vi "PCO_FW_Vers.vi"() -> (0 "PCO_FW_Vers":T2, 1 "PCO_FW_Vers_Raw":T1, 2 "Length":u16, 3 "Raw_Length":u16)   [LabVIEW 2020, in "SDK.lvlib" / "Structures.lvlib"]
doc: "Use this template to build a VI to use as a subVI."
uses:
  Structures.lvlib
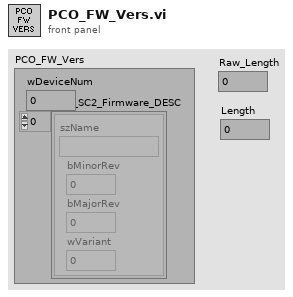
[diagram p1: front panel]
types:
  T1 = cluster{"wDeviceNum":u16, "PCO_SC2_Firmware_DESC":cluster{"PCO_SC2_FW_Desc_Raw":cluster{"szName":cluster{u8, u8, u8, u8, u8, u8, u8, u8, u8, u8, u8, u8, u8, u8, u8, u8}, "bMinorRev":u8, "bMajorRev":u8, "wVariant":u16, "zzwDummy":cluster{u16, u16, u16, u16, u16, u16, u16, u16, u16, u16, u16, u16, u16, u16, u16, u16, u16, u16, u16, u16, u16, u16}}, "PCO_SC2_FW_Desc_Raw":cluster{"szName":cluster{u8, u8, u8, u8, u8, u8, u8, u8, u8, u8, u8, u8, u8, u8, u8, u8}, "bMinorRev":u8, "bMajorRev":u8, "wVariant":u16, "zzwDummy":cluster{u16, u16, u16, u16, u16, u16, u16, u16, u16, u16, u16, u16, u16, u16, u16, u16, u16, u16, u16, u16, u16, u16}}, "PCO_SC2_FW_Desc_Raw":cluster{"szName":cluster{u8, u8, u8, u8, u8, u8, u8, u8, u8, u8, u8, u8, u8, u8, u8, u8}, "bMinorRev":u8, "bMajorRev":u8, "wVariant":u16, "zzwDummy":cluster{u16, u16, u16, u16, u16, u16, u16, u16, u16, u16, u16, u16, u16, u16, u16, u16, u16, u16, u16, u16, u16, u16}}, "PCO_SC2_FW_Desc_Raw":cluster{"szName":cluster{u8, u8, u8, u8, u8, u8, u8, u8, u8, u8, u8, u8, u8, u8, u8, u8}, "bMinorRev":u8, "bMajorRev":u8, "wVariant":u16, "zzwDummy":cluster{u16, u16, u16, u16, u16, u16, u16, u16, u16, u16, u16, u16, u16, u16, u16, u16, u16, u16, u16, u16, u16, u16}}, "PCO_SC2_FW_Desc_Raw":cluster{"szName":cluster{u8, u8, u8, u8, u8, u8, u8, u8, u8, u8, u8, u8, u8, u8, u8, u8}, "bMinorRev":u8, "bMajorRev":u8, "wVariant":u16, "zzwDummy":cluster{u16, u16, u16, u16, u16, u16, u16, u16, u16, u16, u16, u16, u16, u16, u16, u16, u16, u16, u16, u16, u16, u16}}, "PCO_SC2_FW_Desc_Raw":cluster{"szName":cluster{u8, u8, u8, u8, u8, u8, u8, u8, u8, u8, u8, u8, u8, u8, u8, u8}, "bMinorRev":u8, "bMajorRev":u8, "wVariant":u16, "zzwDummy":cluster{u16, u16, u16, u16, u16, u16, u16, u16, u16, u16, u16, u16, u16, u16, u16, u16, u16, u16, u16, u16, u16, u16}}, "PCO_SC2_FW_Desc_Raw":cluster{"szName":cluster{u8, u8, u8, u8, u8, u8, u8, u8, u8, u8, u8, u8, u8, u8, u8, u8}, "bMinorRev":u8, "bMajorRev":u8, "wVariant":u16, "zzwDummy":cluster{u16, u16, u16, u16, u16, u16, u16, u16, u16, u16, u16, u16, u16, u16, u16, u16, u16, u16, u16, u16, u16, u16}}, "PCO_SC2_FW_Desc_Raw":cluster{"szName":cluster{u8, u8, u8, u8, u8, u8, u8, u8, u8, u8, u8, u8, u8, u8, u8, u8}, "bMinorRev":u8, "bMajorRev":u8, "wVariant":u16, "zzwDummy":cluster{u16, u16, u16, u16, u16, u16, u16, u16, u16, u16, u16, u16, u16, u16, u16, u16, u16, u16, u16, u16, u16, u16}}, "PCO_SC2_FW_Desc_Raw":cluster{"szName":cluster{u8, u8, u8, u8, u8, u8, u8, u8, u8, u8, u8, u8, u8, u8, u8, u8}, "bMinorRev":u8, "bMajorRev":u8, "wVariant":u16, "zzwDummy":cluster{u16, u16, u16, u16, u16, u16, u16, u16, u16, u16, u16, u16, u16, u16, u16, u16, u16, u16, u16, u16, u16, u16}}, "PCO_SC2_FW_Desc_Raw":cluster{"szName":cluster{u8, u8, u8, u8, u8, u8, u8, u8, u8, u8, u8, u8, u8, u8, u8, u8}, "bMinorRev":u8, "bMajorRev":u8, "wVariant":u16, "zzwDummy":cluster{u16, u16, u16, u16, u16, u16, u16, u16, u16, u16, u16, u16, u16, u16, u16, u16, u16, u16, u16, u16, u16, u16}}}}
  T2 = cluster{"wDeviceNum":u16, "PCO_SC2_Firmware_DESC":cluster{"szName":string, "bMinorRev":u8, "bMajorRev":u8, "wVariant":u16}[]}
  T3 = cluster{"szName":string, "bMinorRev":u8, "bMajorRev":u8, "wVariant":u16}
  T4 = cluster{"szName":cluster{u8, u8, u8, u8, u8, u8, u8, u8, u8, u8, u8, u8, u8, u8, u8, u8}, "bMinorRev":u8, "bMajorRev":u8, "wVariant":u16, "zzwDummy":cluster{u16, u16, u16, u16, u16, u16, u16, u16, u16, u16, u16, u16, u16, u16, u16, u16, u16, u16, u16, u16, u16, u16}}
  T5 = cluster{"PCO_SC2_FW_Desc_Raw":cluster{"szName":cluster{u8, u8, u8, u8, u8, u8, u8, u8, u8, u8, u8, u8, u8, u8, u8, u8}, "bMinorRev":u8, "bMajorRev":u8, "wVariant":u16, "zzwDummy":cluster{u16, u16, u16, u16, u16, u16, u16, u16, u16, u16, u16, u16, u16, u16, u16, u16, u16, u16, u16, u16, u16, u16}}, "PCO_SC2_FW_Desc_Raw":cluster{"szName":cluster{u8, u8, u8, u8, u8, u8, u8, u8, u8, u8, u8, u8, u8, u8, u8, u8}, "bMinorRev":u8, "bMajorRev":u8, "wVariant":u16, "zzwDummy":cluster{u16, u16, u16, u16, u16, u16, u16, u16, u16, u16, u16, u16, u16, u16, u16, u16, u16, u16, u16, u16, u16, u16}}, "PCO_SC2_FW_Desc_Raw":cluster{"szName":cluster{u8, u8, u8, u8, u8, u8, u8, u8, u8, u8, u8, u8, u8, u8, u8, u8}, "bMinorRev":u8, "bMajorRev":u8, "wVariant":u16, "zzwDummy":cluster{u16, u16, u16, u16, u16, u16, u16, u16, u16, u16, u16, u16, u16, u16, u16, u16, u16, u16, u16, u16, u16, u16}}, "PCO_SC2_FW_Desc_Raw":cluster{"szName":cluster{u8, u8, u8, u8, u8, u8, u8, u8, u8, u8, u8, u8, u8, u8, u8, u8}, "bMinorRev":u8, "bMajorRev":u8, "wVariant":u16, "zzwDummy":cluster{u16, u16, u16, u16, u16, u16, u16, u16, u16, u16, u16, u16, u16, u16, u16, u16, u16, u16, u16, u16, u16, u16}}, "PCO_SC2_FW_Desc_Raw":cluster{"szName":cluster{u8, u8, u8, u8, u8, u8, u8, u8, u8, u8, u8, u8, u8, u8, u8, u8}, "bMinorRev":u8, "bMajorRev":u8, "wVariant":u16, "zzwDummy":cluster{u16, u16, u16, u16, u16, u16, u16, u16, u16, u16, u16, u16, u16, u16, u16, u16, u16, u16, u16, u16, u16, u16}}, "PCO_SC2_FW_Desc_Raw":cluster{"szName":cluster{u8, u8, u8, u8, u8, u8, u8, u8, u8, u8, u8, u8, u8, u8, u8, u8}, "bMinorRev":u8, "bMajorRev":u8, "wVariant":u16, "zzwDummy":cluster{u16, u16, u16, u16, u16, u16, u16, u16, u16, u16, u16, u16, u16, u16, u16, u16, u16, u16, u16, u16, u16, u16}}, "PCO_SC2_FW_Desc_Raw":cluster{"szName":cluster{u8, u8, u8, u8, u8, u8, u8, u8, u8, u8, u8, u8, u8, u8, u8, u8}, "bMinorRev":u8, "bMajorRev":u8, "wVariant":u16, "zzwDummy":cluster{u16, u16, u16, u16, u16, u16, u16, u16, u16, u16, u16, u16, u16, u16, u16, u16, u16, u16, u16, u16, u16, u16}}, "PCO_SC2_FW_Desc_Raw":cluster{"szName":cluster{u8, u8, u8, u8, u8, u8, u8, u8, u8, u8, u8, u8, u8, u8, u8, u8}, "bMinorRev":u8, "bMajorRev":u8, "wVariant":u16, "zzwDummy":cluster{u16, u16, u16, u16, u16, u16, u16, u16, u16, u16, u16, u16, u16, u16, u16, u16, u16, u16, u16, u16, u16, u16}}, "PCO_SC2_FW_Desc_Raw":cluster{"szName":cluster{u8, u8, u8, u8, u8, u8, u8, u8, u8, u8, u8, u8, u8, u8, u8, u8}, "bMinorRev":u8, "bMajorRev":u8, "wVariant":u16, "zzwDummy":cluster{u16, u16, u16, u16, u16, u16, u16, u16, u16, u16, u16, u16, u16, u16, u16, u16, u16, u16, u16, u16, u16, u16}}, "PCO_SC2_FW_Desc_Raw":cluster{"szName":cluster{u8, u8, u8, u8, u8, u8, u8, u8, u8, u8, u8, u8, u8, u8, u8, u8}, "bMinorRev":u8, "bMajorRev":u8, "wVariant":u16, "zzwDummy":cluster{u16, u16, u16, u16, u16, u16, u16, u16, u16, u16, u16, u16, u16, u16, u16, u16, u16, u16, u16, u16, u16, u16}}}
  T6 = cluster{"szName":string, "bMinorRev":u8, "bMajorRev":u8, "wVariant":u16}[]
  T7 = cluster{"wDeviceNum":u16, cluster{"szName":string, "bMinorRev":u8, "bMajorRev":u8, "wVariant":u16}[]}
  T8 = cluster{"wDeviceNum":u16, cluster{"PCO_SC2_FW_Desc_Raw":cluster{"szName":cluster{u8, u8, u8, u8, u8, u8, u8, u8, u8, u8, u8, u8, u8, u8, u8, u8}, "bMinorRev":u8, "bMajorRev":u8, "wVariant":u16, "zzwDummy":cluster{u16, u16, u16, u16, u16, u16, u16, u16, u16, u16, u16, u16, u16, u16, u16, u16, u16, u16, u16, u16, u16, u16}}, "PCO_SC2_FW_Desc_Raw":cluster{"szName":cluster{u8, u8, u8, u8, u8, u8, u8, u8, u8, u8, u8, u8, u8, u8, u8, u8}, "bMinorRev":u8, "bMajorRev":u8, "wVariant":u16, "zzwDummy":cluster{u16, u16, u16, u16, u16, u16, u16, u16, u16, u16, u16, u16, u16, u16, u16, u16, u16, u16, u16, u16, u16, u16}}, "PCO_SC2_FW_Desc_Raw":cluster{"szName":cluster{u8, u8, u8, u8, u8, u8, u8, u8, u8, u8, u8, u8, u8, u8, u8, u8}, "bMinorRev":u8, "bMajorRev":u8, "wVariant":u16, "zzwDummy":cluster{u16, u16, u16, u16, u16, u16, u16, u16, u16, u16, u16, u16, u16, u16, u16, u16, u16, u16, u16, u16, u16, u16}}, "PCO_SC2_FW_Desc_Raw":cluster{"szName":cluster{u8, u8, u8, u8, u8, u8, u8, u8, u8, u8, u8, u8, u8, u8, u8, u8}, "bMinorRev":u8, "bMajorRev":u8, "wVariant":u16, "zzwDummy":cluster{u16, u16, u16, u16, u16, u16, u16, u16, u16, u16, u16, u16, u16, u16, u16, u16, u16, u16, u16, u16, u16, u16}}, "PCO_SC2_FW_Desc_Raw":cluster{"szName":cluster{u8, u8, u8, u8, u8, u8, u8, u8, u8, u8, u8, u8, u8, u8, u8, u8}, "bMinorRev":u8, "bMajorRev":u8, "wVariant":u16, "zzwDummy":cluster{u16, u16, u16, u16, u16, u16, u16, u16, u16, u16, u16, u16, u16, u16, u16, u16, u16, u16, u16, u16, u16, u16}}, "PCO_SC2_FW_Desc_Raw":cluster{"szName":cluster{u8, u8, u8, u8, u8, u8, u8, u8, u8, u8, u8, u8, u8, u8, u8, u8}, "bMinorRev":u8, "bMajorRev":u8, "wVariant":u16, "zzwDummy":cluster{u16, u16, u16, u16, u16, u16, u16, u16, u16, u16, u16, u16, u16, u16, u16, u16, u16, u16, u16, u16, u16, u16}}, "PCO_SC2_FW_Desc_Raw":cluster{"szName":cluster{u8, u8, u8, u8, u8, u8, u8, u8, u8, u8, u8, u8, u8, u8, u8, u8}, "bMinorRev":u8, "bMajorRev":u8, "wVariant":u16, "zzwDummy":cluster{u16, u16, u16, u16, u16, u16, u16, u16, u16, u16, u16, u16, u16, u16, u16, u16, u16, u16, u16, u16, u16, u16}}, "PCO_SC2_FW_Desc_Raw":cluster{"szName":cluster{u8, u8, u8, u8, u8, u8, u8, u8, u8, u8, u8, u8, u8, u8, u8, u8}, "bMinorRev":u8, "bMajorRev":u8, "wVariant":u16, "zzwDummy":cluster{u16, u16, u16, u16, u16, u16, u16, u16, u16, u16, u16, u16, u16, u16, u16, u16, u16, u16, u16, u16, u16, u16}}, "PCO_SC2_FW_Desc_Raw":cluster{"szName":cluster{u8, u8, u8, u8, u8, u8, u8, u8, u8, u8, u8, u8, u8, u8, u8, u8}, "bMinorRev":u8, "bMajorRev":u8, "wVariant":u16, "zzwDummy":cluster{u16, u16, u16, u16, u16, u16, u16, u16, u16, u16, u16, u16, u16, u16, u16, u16, u16, u16, u16, u16, u16, u16}}, "PCO_SC2_FW_Desc_Raw":cluster{"szName":cluster{u8, u8, u8, u8, u8, u8, u8, u8, u8, u8, u8, u8, u8, u8, u8, u8}, "bMinorRev":u8, "bMajorRev":u8, "wVariant":u16, "zzwDummy":cluster{u16, u16, u16, u16, u16, u16, u16, u16, u16, u16, u16, u16, u16, u16, u16, u16, u16, u16, u16, u16, u16, u16}}}}
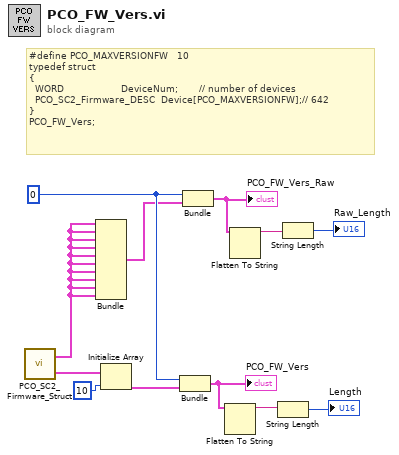
[diagram p0: block diagram]
diagram:
  w3 = u16 0 ("wDeviceNum")
  # "#define PCO_MAXVERSIONFW   10\ntypedef struct\n{\n  WORD                   DeviceNum;       // number of devices\n  PCO_SC2_Firmware_DESC  Device[PCO_MAXVERSIONFW];// 642\n}\nPCO_FW_Vers;"
  n1 = call "PCO_SC2_Firmware_Struct.vi"() -> ("PCO_SC2_FW_Desc"=w5:T3, "PCO_SC2_FW_Desc_Raw"=w1:T4)  [unwired: 4 in, 2 out]
  n2 = Bundle("PCO_SC2_FW_Desc_Raw"=w1, "PCO_SC2_FW_Desc_Raw"=w1, "PCO_SC2_FW_Desc_Raw"=w1, "PCO_SC2_FW_Desc_Raw"=w1, "PCO_SC2_FW_Desc_Raw"=w1, "PCO_SC2_FW_Desc_Raw"=w1, "PCO_SC2_FW_Desc_Raw"=w1, "PCO_SC2_FW_Desc_Raw"=w1, "PCO_SC2_FW_Desc_Raw"=w1, "PCO_SC2_FW_Desc_Raw"=w1) -> (w2:T5)  [unwired: 1 in]
  n3 = Initialize Array(w5, 10 ("dimension size")) -> (w4:T6)
  n4 = Bundle("wDeviceNum"=w3, w4) -> (w8:T7)  [unwired: 1 in]
  "PCO_FW_Vers" <- w8
  n5 = Bundle("wDeviceNum"=w3, w2) -> (w7:T8)  [unwired: 1 in]
  "PCO_FW_Vers_Raw" <- w7
  n6 = Flatten To String(anything=w8) -> (data string=w10:string)  [unwired: 3 in, 2 out]
  n7 = Flatten To String(anything=w7) -> (data string=w12:string)  [unwired: 3 in, 2 out]
  n8 = String Length(string=w10) -> (length=→"Length":i32)
  n9 = String Length(string=w12) -> (length=→"Raw_Length":i32)
